vi "pockelscontrol_w_blanking_roMD.vi"() -> ()   [LabVIEW 2012]
doc: "SciScan 1.2 160622"
uses:
  <vilib>/Utility/VariantDataType/Type.ctl
  Custom Controls/Pockels data structure (for laser power control).ctl
  <vilib>/DAQmx/write.llb/DAQmx Write (Analog 1D DBL 1Chan NSamp).vi
  <vilib>/DAQmx/write.llb/DAQmx Write (Analog 2D DBL NChan NSamp).vi
  GFG/GFGfpRefGet.vi
  <vilib>/DAQmx/miscellaneous.llb/DAQmx Fill In Error Info.vi
  GFG/GFGnumericGet.vi
  GFG/GFGbooleanGet.vi
  GFG/GFGstringGet.vi
  GFG/GFG library.lvlib
  <vilib>/Utility/VariantDataType/VariantType.lvlib
panel:
  out "error out 3":errorcluster
  out "error out 2":errorcluster
  out "error out":errorcluster
  out "Source VI":string
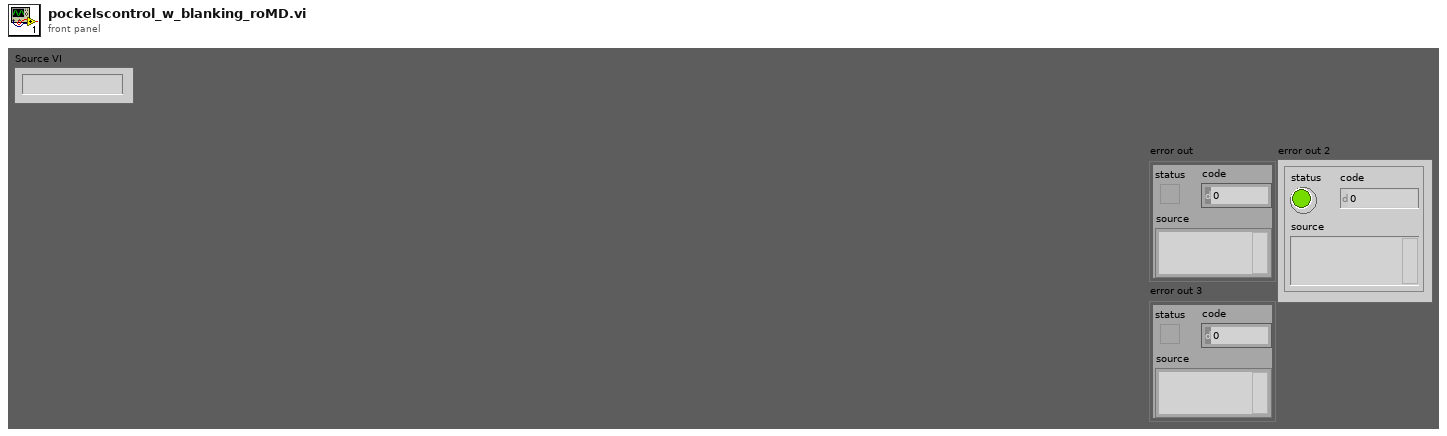
[diagram p1: front panel]
types:
  T1 = enum8{"Enabled", "Disabled", "Disabled and Grayed Out"}
  T2 = cluster{"WaveformChartRef":refnum<vi>, "DigitalRef":refnum<vi>, "ArrayRef":refnum<vi>, "TabControlRef":refnum<vi>, "EnumRef":refnum<vi>, "RingRef":refnum<vi>, "BooleanRef":refnum<vi>, "KnobRef":refnum<vi>, "SlideRef":refnum<vi>, "PathRef":refnum<vi>, "StringRef":refnum<vi>, "ComboBox":refnum<vi>, "WaveformGraphRef":refnum<vi>}
  T3 = enum16{"Left Button", "Center Button", "Right Button", "Window Close"}
  T4 = typedef "Pockels data structure (for laser power control).ctl" = cluster{"DAQmx Task Name (Pockels)":refnum<k21>, "(Sharing Pocekls Card?)YGalvo, Pockels,Piezo":bool[]}
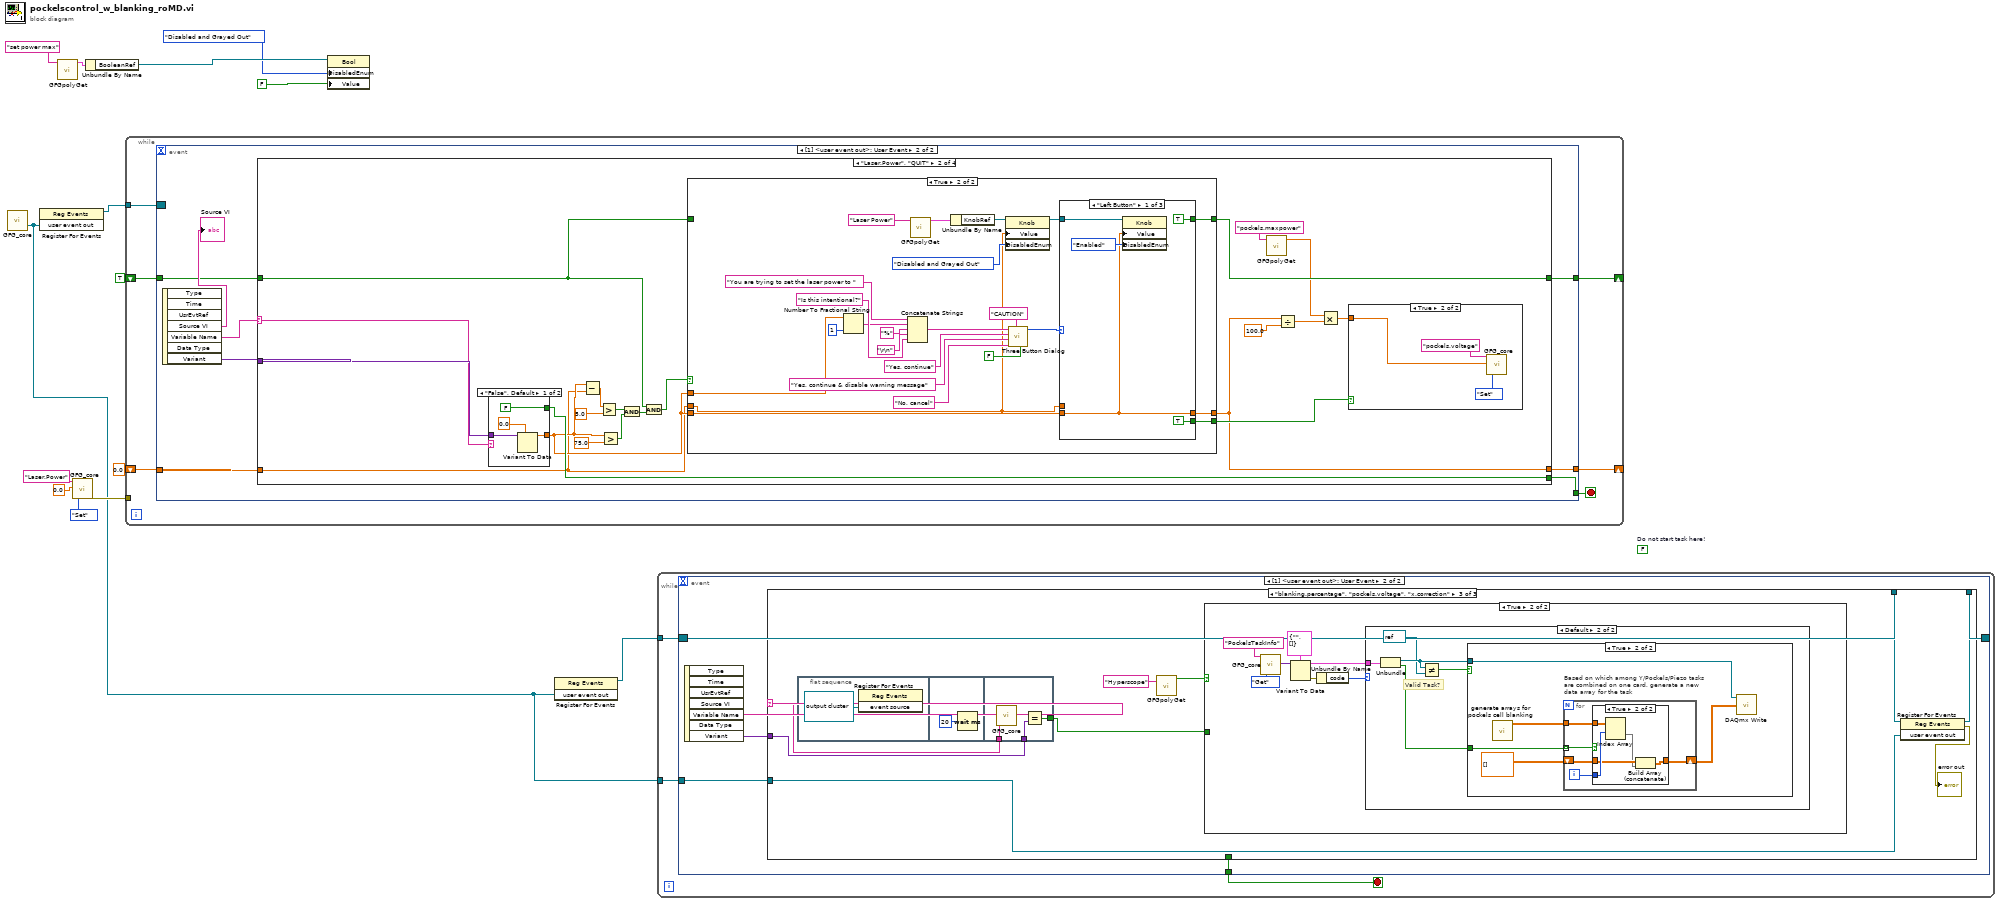
[diagram p0: block diagram]
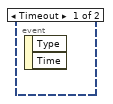
[diagram p2: hidden frame]
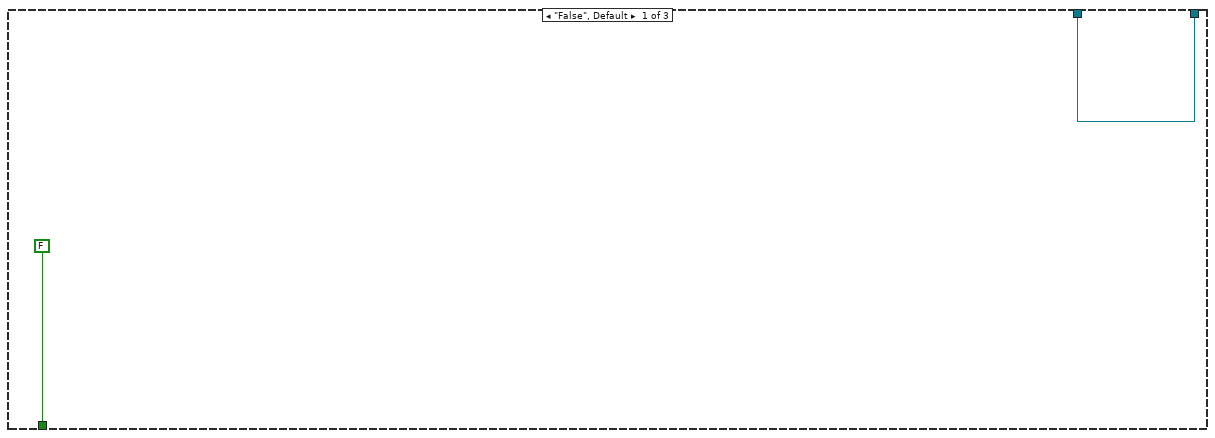
[diagram p3: hidden frame]
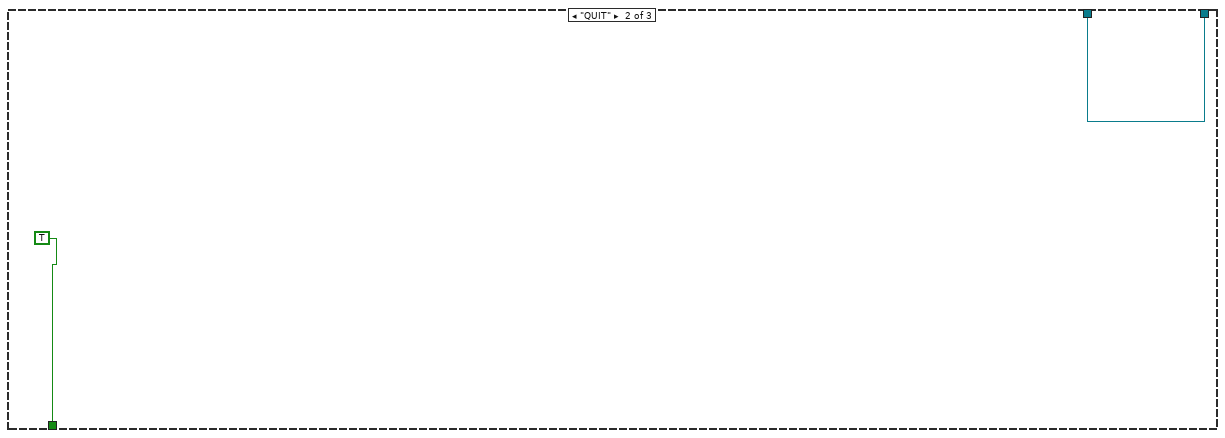
[diagram p4: hidden frame]
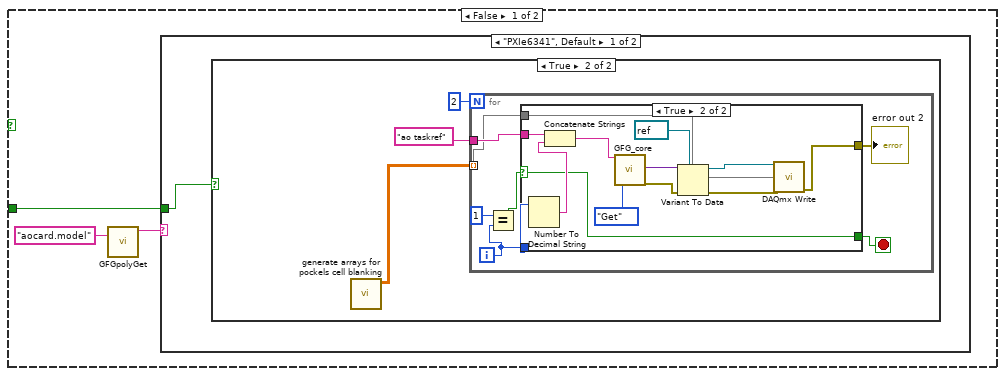
[diagram p5: hidden frame]
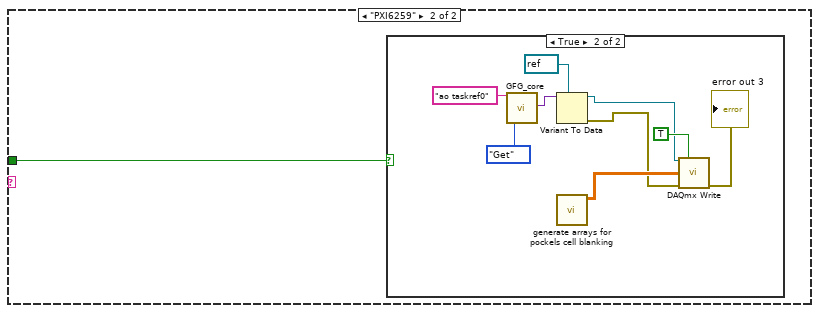
[diagram p8: hidden frame]
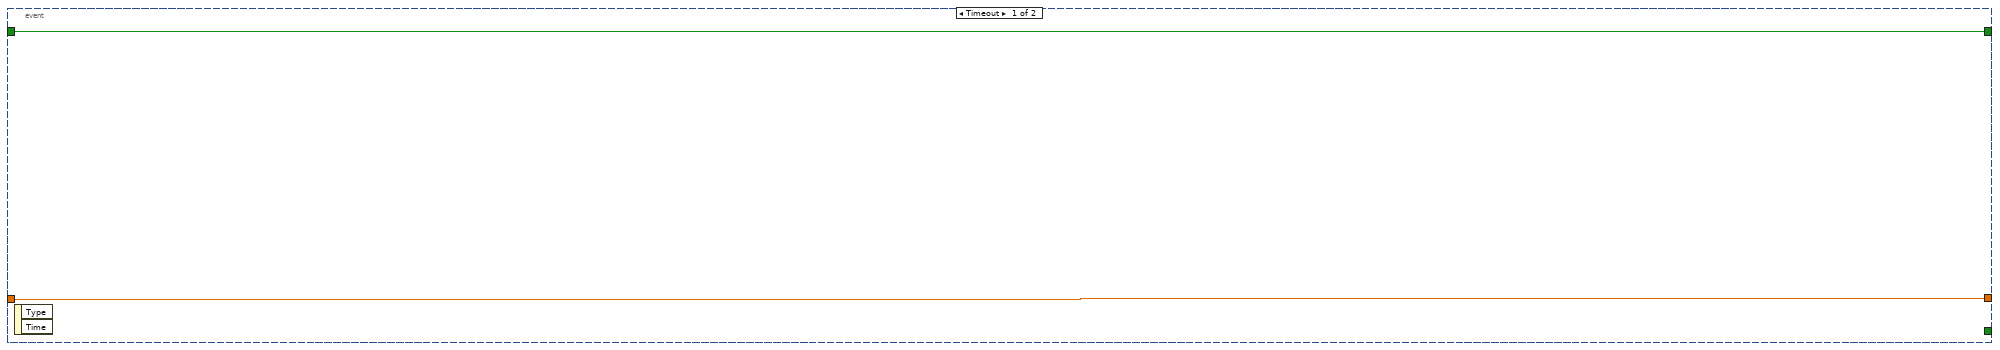
[diagram p13: hidden frame]
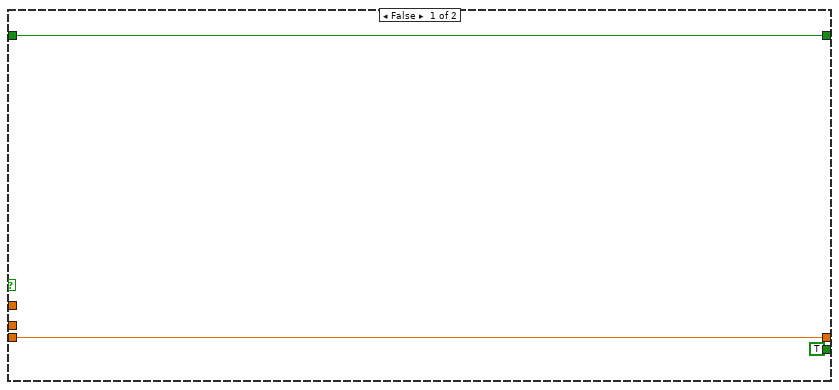
[diagram p15: hidden frame]
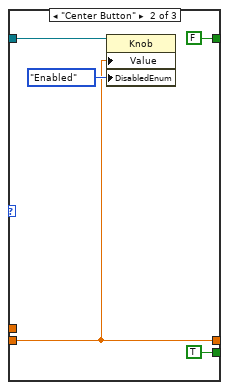
[diagram p16: hidden frame]
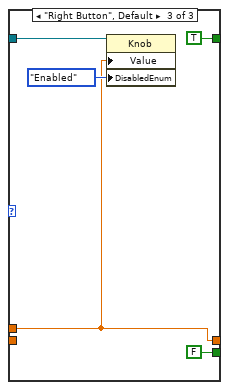
[diagram p17: hidden frame]
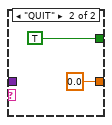
[diagram p19: hidden frame]
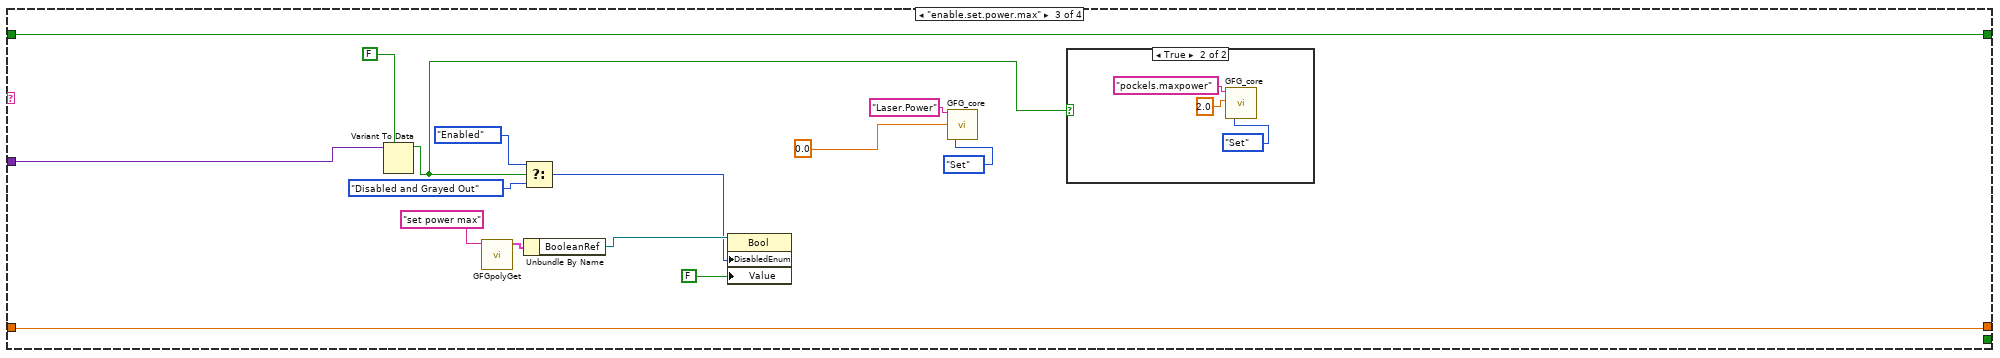
[diagram p20: hidden frame]
diagram:
  (unwired) FALSE  # Do not start task here!
  n1 = call "GFG_core.vi"() -> ("user event out"=w1:refnum<user-event>)  [unwired: 13 in, 6 out]
  n2 = register-events(w1) -> (reference out=w14:refnum<event-registration>)  [unwired: 2 in, 1 out]
  n3 = call-poly "GFGpolyGet.vi"("Variable Name in"="set power max") -> ("output cluster"=w6:T2)  [unwired: 9 in, 1 out]
  n4 = call "GFG_core.vi"("Variable Name in"="Laser.Power", "Variant in"=0.0 ("Laser Power"), "Action"=enum16{"Init", "Set", "Get"}."Set") -> ("error out"=w2:errorcluster)  [unwired: 10 in, 6 out]
  n5 = Unbundle By Name(w6) -> ("BooleanRef"=w7:refnum<vi>)
  n6 = while {
    tunnel: w14 -> [w20]
    shift-right: [w18] -> _
    shift-left: 0.0 ("Laser Power") -> [w17]
    shift-right: [w16] -> _
    shift-left: TRUE -> [w15]
    tunnel: w2 -> [_]
    stop <- w19 stop-if-true
    n7 = event shown="[1] <user event out>: User Event" {
      selector: w20 -> [_ _]
      dyn-events: _ -> [_ _]
      timeout: _ -> [_ _]
      tunnel: [_ w27] -> w19
      tunnel: [w22 w26] -> w18
      tunnel: w17 -> [w22 w25]
      tunnel: [w21 w24] -> w16
      tunnel: w15 -> [w21 w23]
      event Timeout {
        n8 = event-data() -> ()  [unwired: 1 in, 2 out]
      }
      event User Event {
        n9 = event-data() -> ("Source VI"=→"Source VI":string, "Variable Name"=w30:string, "Variant"=w29:variant)  [unwired: 1 in, 4 out]
        n10 = case shown="\"Laser.Power\", \"QUIT\"" w30 {
          selector: w30 -> [_ w52 _ _]
          tunnel: w29 -> [_ w53 w111 _]
          tunnel: [_ w51 _ _] -> w27
          tunnel: [w32 w41 w116 w137] -> w26
          tunnel: w25 -> [w32 w38 w116 w137]
          tunnel: [w31 w44 w115 w136] -> w24
          tunnel: w23 -> [w31 w42 w115 w136]
          frame "False", Default {
          }
          frame "Laser.Power", "QUIT" {
            n11 = case shown="\"False\", Default" w52 {
              tunnel: w53 -> [w102 _]
              tunnel: [w101 0.0 ("Laser Power")] -> w39
              tunnel: [FALSE TRUE] -> w51
              frame "False", Default {
                n12 = Variant To Data(type=0.0 ("Laser Power"), Variant=w102) -> (data=w101:dbl)  [unwired: 1 in, 1 out]
              }
              frame "QUIT" {
              }
            }
            n13 = Subtract(x=w39, y=w38) -> (x-y=w37:dbl)
            n14 = Greater?(x=w37, y=5.0) -> (0:w35:bool)
            n15 = Greater?(x=w39, y=75.0) -> (0:w47:bool)
            n16 = And(x=w35, y=w47) -> (x .and. y?=w40:bool)
            n17 = And(x=w42, y=w40) -> (x .and. y?=w43:bool)
            n18 = case shown="True" w43 {
              tunnel: [TRUE w74] -> w45
              tunnel: [w55 w73] -> w44
              tunnel: w42 -> [w55 _]
              tunnel: w38 -> [_ w61]
              tunnel: w39 -> [_ w71]
              tunnel: w39 -> [w54 w62]
              tunnel: [w54 w57] -> w41
              frame False {
              }
              frame True {
                n19 = Number To Fractional String(number=w71, precision (6)=i16 1) -> (F-format string=w60:string)  [unwired: 2 in]
                n20 = Concatenate Strings("You are trying to set the laser power to " ("message"), w60, "%" ("string"), "\r\n", "Is this intentional?" ("string")) -> (w68:string)
                n21 = call-poly "GFGpolyGet.vi"("Variable Name in"="Laser Power") -> ("output cluster"=w66:T2)  [unwired: 9 in, 1 out]
                n22 = Unbundle By Name(w66) -> ("KnobRef"=w65:refnum<vi>)
                n23 = property class="Knob"(reference=w65, "Value"=w61, "DisabledEnum"=T1."Disabled and Grayed Out" ("Disabled")) -> (reference out=w63:refnum<vi>)  [unwired: 1 in, 1 out]
                n24 = call <vilib>:"Three Button Dialog.vi"("Allow user to close window? (TRUE)"=FALSE, "Window Title (\"\")"="CAUTION" ("Window Title (\"\")"), "Right Button Text (\"Cancel\")"="No, cancel" ("Right Button Text (\"Cancel\")"), "Center Button Text (\"No\")"="Yes, continue & disable warning message" ("Center Button Text (\"No\")"), "Left Button Text (\"Yes\")"="Yes, continue" ("Left Button Text (\"Yes\")"), "message"=w68) -> ("Which Button?"=w75:T3)  [unwired: 5 in]
                n25 = case shown="\"Left Button\"" w75 {
                  tunnel: [TRUE TRUE FALSE] -> w74
                  tunnel: [TRUE FALSE TRUE] -> w73
                  tunnel: w63 -> [w82 w87 w92]
                  tunnel: w62 -> [w81 w86 _]
                  tunnel: w61 -> [_ _ w91]
                  tunnel: [w81 w86 w91] -> w57
                  frame "Left Button" {
                    n26 = property class="Knob"(reference=w82, "Value"=w81, "DisabledEnum"=T1."Enabled" ("Disabled")) -> ()  [unwired: 1 in, 2 out]
                  }
                  frame "Center Button" {
                    n27 = property class="Knob"(reference=w87, "Value"=w86, "DisabledEnum"=T1."Enabled" ("Disabled")) -> ()  [unwired: 1 in, 2 out]
                  }
                  frame "Right Button", Default {
                    n28 = property class="Knob"(reference=w92, "Value"=w91, "DisabledEnum"=T1."Enabled" ("Disabled")) -> ()  [unwired: 1 in, 2 out]
                  }
                }
              }
            }
            n29 = call-poly "GFGpolyGet.vi"("Variable Name in"="pockels.maxpower") -> ("Numeric"=w33:dbl)  [unwired: 8 in, 2 out]
            n30 = Divide(x=w41, y=100.0 ("x")) -> (x/y=w50:dbl)
            n31 = Multiply(x=w33, y=w50) -> (x*y=w48:dbl)
            n32 = case shown="True" w45 {
              tunnel: w48 -> [_ w96]
              frame False {
              }
              frame True {
                n33 = call "GFG_core.vi"("Variable Name in"="pockels.voltage", "Variant in"=w96, "Action"=enum16{"Init", "Set", "Get"}."Set") -> ()  [unwired: 10 in, 7 out]
              }
            }
          }
          frame "enable.set.power.max" {
            n34 = Variant To Data(type=FALSE, Variant=w111) -> (data=w106:bool)  [unwired: 1 in, 1 out]
            n35 = call-poly "GFGpolyGet.vi"("Variable Name in"="set power max") -> ("output cluster"=w118:T2)  [unwired: 9 in, 1 out]
            n36 = Select(t=T1."Enabled" ("Disabled"), s=w106, f=T1."Disabled and Grayed Out" ("Disabled")) -> (s? t:f=w107:T1)
            n37 = Unbundle By Name(w118) -> ("BooleanRef"=w117:refnum<vi>)
            n38 = property class="Bool"(reference=w117, "DisabledEnum"=w107, "Value"=FALSE) -> ()  [unwired: 1 in, 2 out]
            n39 = call "GFG_core.vi"("Variable Name in"="Laser.Power", "Variant in"=0.0 ("Laser Power"), "Action"=enum16{"Init", "Set", "Get"}."Set") -> ()  [unwired: 10 in, 7 out]
            n40 = case shown="True" w106 {
              frame False {
              }
              frame True {
                n41 = call "GFG_core.vi"("Variable Name in"="pockels.maxpower", "Variant in"=2.0 ("Laser Power"), "Action"=enum16{"Init", "Set", "Get"}."Set") -> ()  [unwired: 10 in, 7 out]
              }
            }
          }
          frame "set.power.max" {
            n42 = flat-sequence {
              tunnel: [w144] -> w132
              tunnel: [w143] -> w128
              frame #0 {
                n43 = call-poly "GFGpolyGet.vi"("Variable Name in"="Laser Power") -> ("error out"=w143:errorcluster, "Numeric"=w144:dbl)  [unwired: 8 in, 1 out]
              }
            }
            n44 = Divide(x=w132, y=100.0 ("x")) -> (x/y=w131:dbl)
            n45 = disable-structure shown="Disabled" {
              frame Disabled {
                n46 = call-poly "GFGpolyGet.vi"("Variable Name in"="set power max") -> ("output cluster"=w149:T2)  [unwired: 9 in, 1 out]
                n47 = Unbundle By Name(w149) -> ("BooleanRef"=w148:refnum<vi>)
                n48 = property class="Bool"(reference=w148, "DisabledEnum"=T1."Disabled and Grayed Out" ("Disabled"), "Value"=FALSE) -> ()  [unwired: 1 in, 2 out]
              }
              frame Enabled {
              }
            }
            n49 = Multiply(x=2.0 ("Laser Power"), y=w131) -> (x*y=w129:dbl)
            n50 = call "GFG_core.vi"("Variable Name in"="pockels.maxpower", "Variant in"=w129, "error in (no error)"=w128, "Action"=enum16{"Init", "Set", "Get"}."Set") -> ("error out"=w127:errorcluster)  [unwired: 9 in, 6 out]
            n51 = disable-structure shown="Enabled" {
              disable-tunnel: w127 -> [w139 _]
              disable-tunnel: [w138 _] -> w124
              frame Enabled {
                n52 = call "GFG_core.vi"("Variable Name in"="Laser.Power", "Variant in"=0.0 ("Laser Power"), "error in (no error)"=w139, "Action"=enum16{"Init", "Set", "Get"}."Set") -> ("error out"=w138:errorcluster)  [unwired: 9 in, 6 out]
              }
              frame Disabled {
              }
            }
            n53 = call "GFG_core.vi"("Variable Name in"="enable.set.power.max", "Variant in"=FALSE, "error in (no error)"=w124, "Action"=enum16{"Init", "Set", "Get"}."Set") -> ()  [unwired: 9 in, 7 out]
          }
        }
      }
    }
  }
  n54 = property class="Bool"(reference=w7, "DisabledEnum"=T1."Disabled and Grayed Out" ("Disabled"), "Value"=FALSE) -> ()  [unwired: 1 in, 2 out]
  n55 = register-events(w1) -> (reference out=w3:refnum<event-registration>)  [unwired: 2 in, 1 out]
  n56 = while {
    tunnel: w3 -> [w153]
    tunnel: w1 -> [w151]
    stop <- w152 stop-if-true
    n57 = event shown="[1] <user event out>: User Event" {
      selector: w153 -> [_ w156]
      dyn-events: [_ w155] -> _
      timeout: _ -> [_ _]
      tunnel: [_ w158] -> w152
      tunnel: w151 -> [_ w154]
      event Timeout {
        n58 = event-data() -> ()  [unwired: 1 in, 2 out]
      }
      event User Event {
        n59 = event-data() -> ("Variable Name"=w159:string, "Variant"=w157:variant)  [unwired: 1 in, 5 out]
        n60 = case shown="\"blanking.percentage\", \"pockels.voltage\", \"x.correction\"" w159 {
          selector: w159 -> [_ _ w171]
          tunnel: [FALSE TRUE _] -> w158
          tunnel: w157 -> [_ _ w170]
          tunnel: w156 -> [w160 w162 w168]
          tunnel: [w160 w162 w167] -> w155
          tunnel: w154 -> [_ _ w169]
          frame "False", Default {
          }
          frame "QUIT" {
          }
          frame "blanking.percentage", "pockels.voltage", "x.correction" {
            n61 = flat-sequence {
              tunnel: w171 -> [w243]
              tunnel: [w241] -> w172
              tunnel: w170 -> [w240]
              frame #0 {
                n62 = register-events(refnum<user-event> refnum ("event source")) -> ()  [unwired: 2 in, 2 out]
              }
              frame #1 {
                n63 = Wait (ms)(milliseconds to wait=u32 20) -> ()  [unwired: 1 out]
              }
              frame #2 {
                n64 = call "GFG_core.vi"("Variable Name in"=w243) -> ("Variant Out"=w242:variant)  [unwired: 12 in, 6 out]
                n65 = Equal?(x=w242, y=w240) -> (x = y?=w241:bool)
              }
            }
            n66 = call-poly "GFGpolyGet.vi"("Variable Name in"="Hyperscope") -> ("Boolean Value OUT"=w164:bool)  [unwired: 9 in, 1 out]
            n67 = case shown="True" w164 {
              tunnel: w172 -> [w175 _]
              frame False {
                n68 = call-poly "GFGpolyGet.vi"("Variable Name in"="aocard.model") -> ("String"=w173:string)  [unwired: 9 in, 1 out]
                n69 = case shown="\"PXIe6341\", Default" w173 {
                  tunnel: w175 -> [w176 w200]
                  frame "PXIe6341", Default {
                    n70 = case shown="True" w176 {
                      frame False {
                      }
                      frame True {
                        n71 = call "generate arrays for pockels cell blanking.vi"() -> ("Array"=w177:dbl[][])  [unwired: 11 in]
                        n72 = for {
                          N: 2 -> [_]
                          tunnel: "ao taskref" ("Variable Name in") -> [w186]
                          tunnel: w177 -> [w185] mode=indexing
                          i -> [w184]
                          stop <- w181 stop-if-true
                          n73 = Equal?(x=1, y=w184) -> (x = y?=w182:bool)
                          n74 = case shown="True" w182 {
                            selector: w182 -> [_ w188]
                            tunnel: w184 -> [_ w198]
                            tunnel: w186 -> [_ w196]
                            tunnel: w185 -> [_ w189]
                            tunnel: [_ w188] -> w181
                            tunnel: [_ w187] -> w180
                            frame False {
                            }
                            frame True {
                              n75 = Number To Decimal String(number=w198) -> (decimal integer string=w197:string)  [unwired: 1 in]
                              n76 = Concatenate Strings(w196, w197) -> (w195:string)
                              n77 = call "GFG_core.vi"("Variable Name in"=w195, "Action"=enum16{"Init", "Set", "Get"}."Get") -> ("Variant Out"=w193:variant, "error out"=w194:errorcluster)  [unwired: 11 in, 5 out]
                              n78 = Variant To Data(error in=w194, type=refnum<k21> refnum ("task out"), Variant=w193) -> (data=w191:refnum<k21>, error out=w190:errorcluster)
                              n79 = call-poly <vilib>:"DAQmx Write.vi"("task/channels in"=w191, "data"=w189, "error in"=w190) -> ("error out"=w187:errorcluster)  [unwired: 10 in, 2 out]
                            }
                          }
                          "error out 2" <- w180
                        }
                      }
                    }
                  }
                  frame "PXI6259" {
                    n80 = case shown="True" w200 {
                      frame False {
                      }
                      frame True {
                        n81 = call "GFG_core.vi"("Variable Name in"="ao taskref0", "Action"=enum16{"Init", "Set", "Get"}."Get") -> ("Variant Out"=w208:variant)  [unwired: 11 in, 6 out]
                        n82 = Variant To Data(type=refnum<k21> refnum ("task out"), Variant=w208) -> (data=w203:refnum<k21>, error out=w202:errorcluster)  [unwired: 1 in]
                        n83 = call "generate arrays for pockels cell blanking.vi"() -> ("Array"=w204:dbl[][])  [unwired: 11 in]
                        n84 = call-poly <vilib>:"DAQmx Write.vi"("task/channels in"=w203, "auto start"=TRUE, "data"=w204, "error in"=w202) -> ("error out"=→"error out 3":errorcluster)  [unwired: 9 in, 2 out]
                      }
                    }
                  }
                }
              }
              frame True {
                n85 = call "GFG_core.vi"("Variable Name in"="PockelsTaskInfo", "Action"=enum16{"Init", "Set", "Get"}."Get") -> ("Variant Out"=w214:variant)  [unwired: 11 in, 6 out]
                n86 = Variant To Data(type=T4 {"DAQmx Task Name (Pockels)"="", "(Sharing Pocekls Card?)YGalvo, Pockels,Piezo"=[]} ("Pockels Data Structure (for Laser Power Control)"), Variant=w214) -> (data=w212:T4, error out=w211:errorcluster)  [unwired: 1 in]
                n87 = Unbundle By Name(w211) -> ("code"=w210:i32)
                n88 = case shown="Default" w210 {
                  tunnel: w212 -> [_ w221]
                  frame 91 {
                    # "Error 91 Occurs when Task has not yet been configured - eg., during startup"
                  }
                  frame Default {
                    # "Valid Task?"
                    n89 = Unbundle(w221) -> ("DAQmx Task Name (Pockels)"=w219:refnum<k21>, "(Sharing Pocekls Card?)YGalvo, Pockels,Piezo"=w217:bool[])
                    n90 = Not Equal?(x=w219, y=refnum<k21> refnum ("DAQmx Task Name (Pockels)")) -> (x != y?=w220:bool)
                    n91 = case shown="True" w220 {
                      tunnel: w219 -> [_ w226]
                      tunnel: w217 -> [_ w224]
                      frame False {
                      }
                      frame True {
                        n92 = call "generate arrays for pockels cell blanking.vi"() -> ("Array"=w222:dbl[][])  [unwired: 11 in]
                        n93 = for "Based on which among Y/Pockels/Piezo tasks are combined on one card, generate a new data array for the task" {
                          tunnel: w222 -> [w230]
                          tunnel: w224 -> [w231] mode=indexing
                          shift-right: [w227] -> w223
                          shift-left: dbl[][] [] ("Array") -> [w228]
                          i -> [w229]
                          n94 = case shown="True" w231 {
                            tunnel: w230 -> [_ w237]
                            tunnel: w229 -> [_ w236]
                            tunnel: w228 -> [w232 w235]
                            tunnel: [w232 w233] -> w227
                            frame False {
                            }
                            frame True {
                              n95 = Index Array(array=w237, index (row)=w236) -> (element=w234:dbl[])  [unwired: 1 in]
                              n96 = Build Array (concatenate)(w235, w234) -> (w233:dbl[][])
                            }
                          }
                        }
                        n97 = call-poly <vilib>:"DAQmx Write.vi"("task/channels in"=w226, "data"=w223) -> ()  [unwired: 11 in, 3 out]
                      }
                    }
                  }
                }
              }
            }
            n98 = register-events(reference=w168, w169) -> (reference out=w167:refnum<event-registration>, error out=→"error out":errorcluster)  [unwired: 1 in]
          }
        }
      }
    }
  }
